vi "Main.vi"(8 "error in (no error)":T1) -> (0 "error out":T1)   [LabVIEW 2019, in "Log.lvlib"]
doc: "Logs commands and errors in\nlog file"
uses:
  Log.lvlib
  module data.ctl
  log module message.ctl
  <vilib>/Field R&D Services/Logger/Type Definitions/Severity.ctl
  681a73ac-a301-4c4f-9af0-9afa4de37740.vi
  Log GV.vi
  SubVIs/Shared/Comm GV.vi
  SubVIs/Shared/System GV.vi
  <vilib>/Field R&D Services/Logger/Support/Manager.vi
  <vilib>/Field R&D Services/Logger/Support/Control State.vi
  SubVIs/Shared/Shared.lvlib
  <vilib>/Field R&D Services/Logger/Field_RnD_Services_Logger_Toolkit.lvlib
panel:
  in  "stop wd":bool
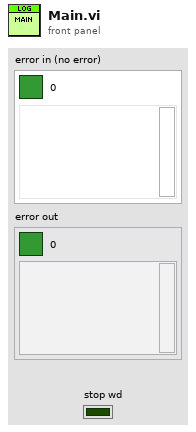
[diagram p1: front panel]
types:
  T1 = cluster{"Boolean Round":bool, "code":i32, "source":string}
  T2 = typedef "Log.lvlib/log module message.ctl" = cluster{"msg":string, "data":string}
  T3 = typedef "Log.lvlib/module data.ctl" = cluster{"dummy":dbl}
  T4 = typedef "Field_RnD_Services_Logger_Toolkit.lvlib/Severity.ctl" = enum16{"Benign", "Warning", "Recoverable", "Fatal"}
  T5 = typedef "CommandResponse communication.lvlib/Status + response + data cluster.ctl" = cluster{"message":string, "response":string, "data":variant}
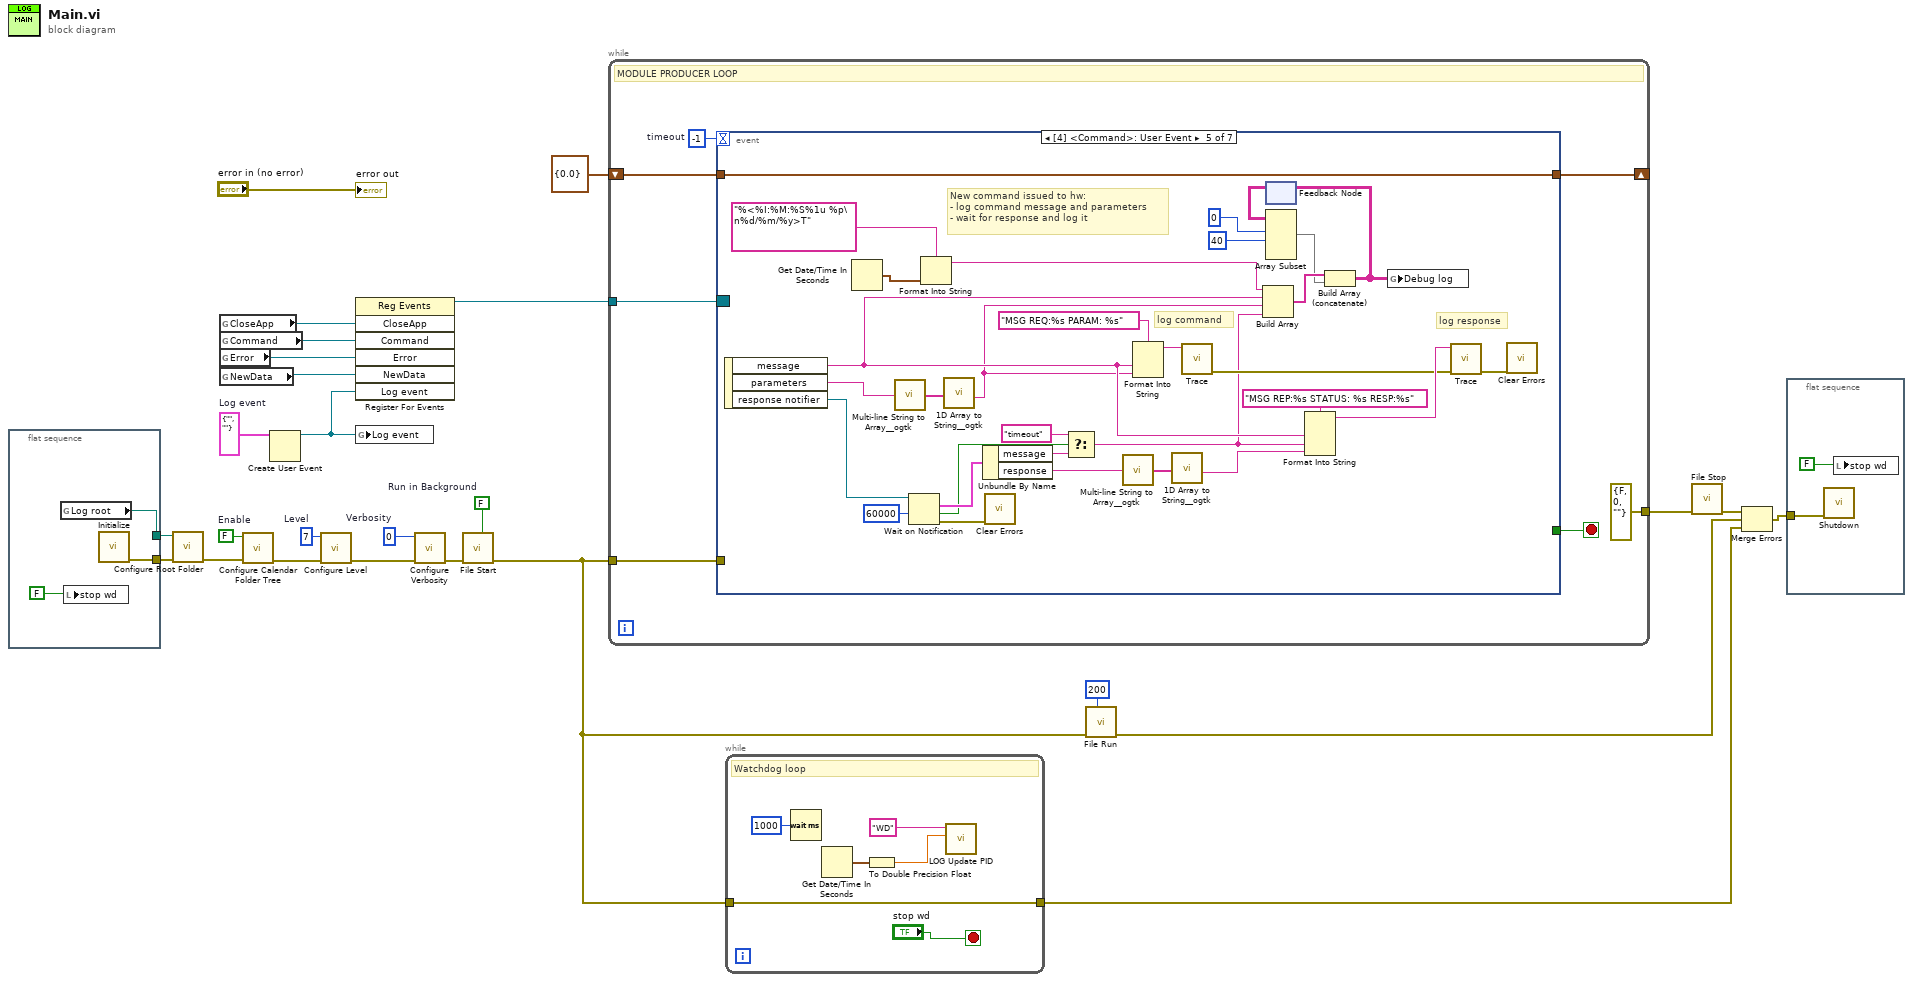
[diagram p0: block diagram]
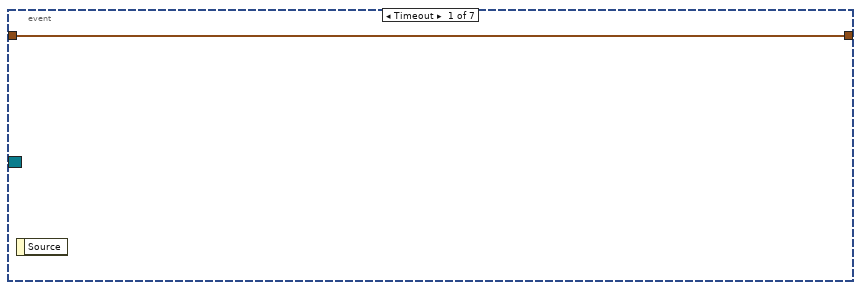
[diagram p2: hidden frame]
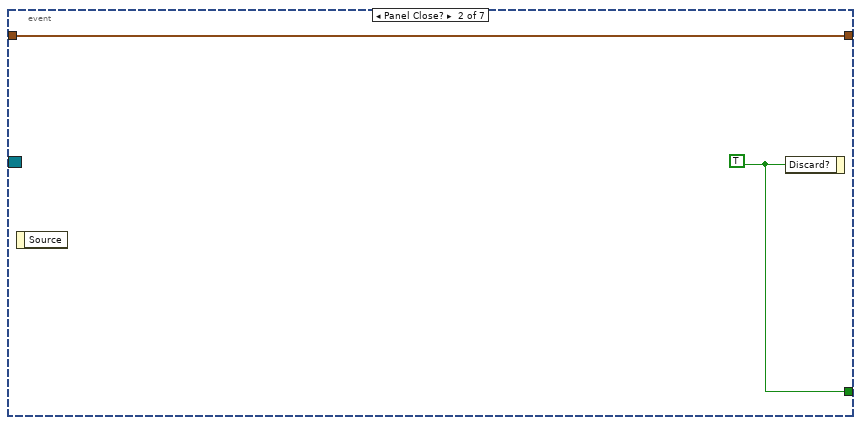
[diagram p3: hidden frame]
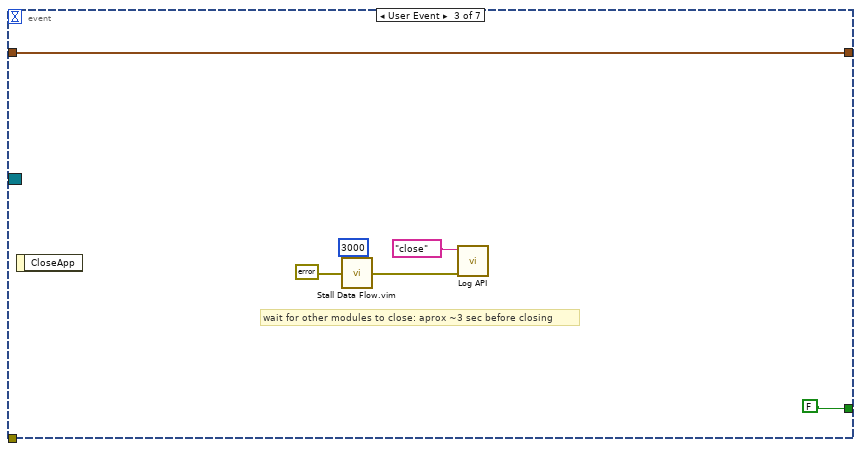
[diagram p4: hidden frame]
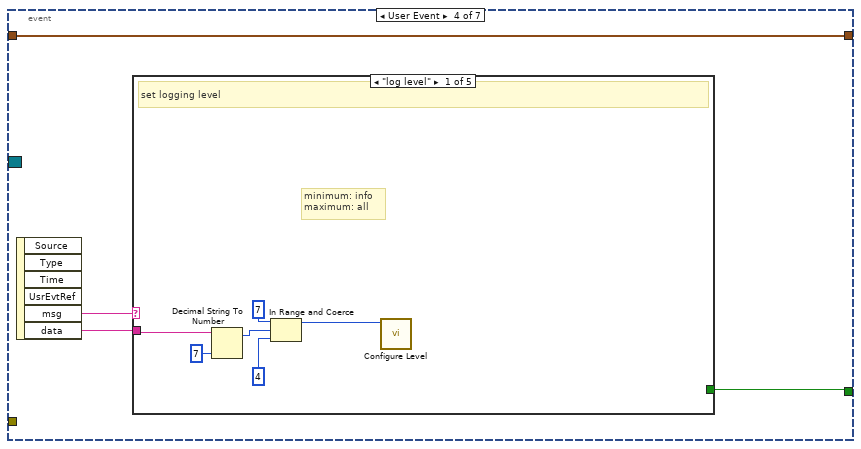
[diagram p5: hidden frame]
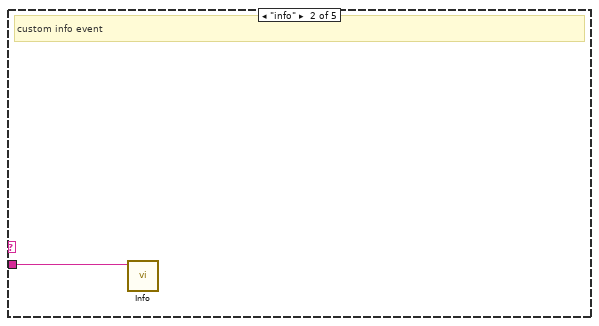
[diagram p6: hidden frame]
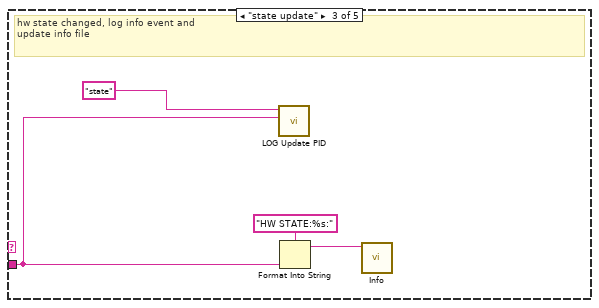
[diagram p7: hidden frame]
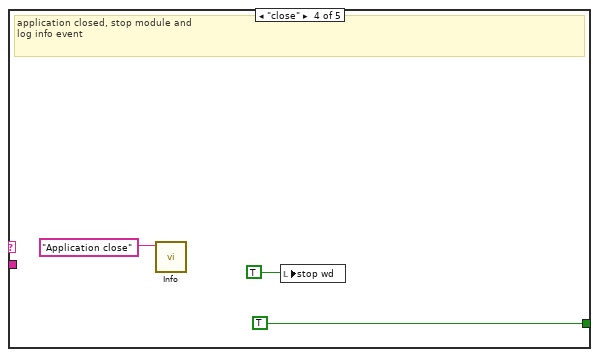
[diagram p8: hidden frame]
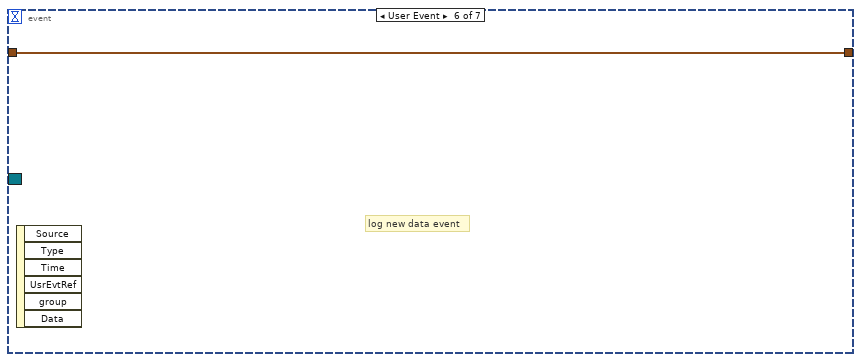
[diagram p10: hidden frame]
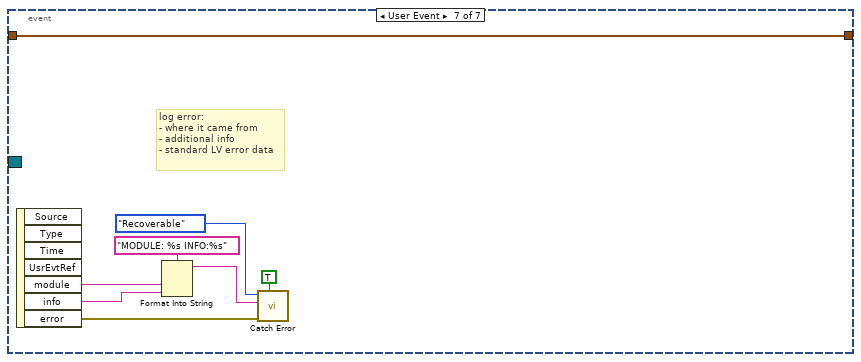
[diagram p11: hidden frame]
diagram:
  w5 = T2 {"msg"="", "data"=""}  # Log event
  w11 = u8 7  # Level
  w13 = FALSE  # Run in Background
  w17 = u8 0  # Verbosity
  w14 = FALSE  # Enable
  n1 = flat-sequence {
    tunnel: [w29] -> w20
    tunnel: [w28] -> w19
    frame #0 {
      n2 = global read "System GV.vi" "Log root"() -> (w28:path)
      n3 = local write "stop wd"(FALSE) -> ()
      n4 = call <vilib>:"Initialize.vi"() -> ("Error Out"=w29:errorcluster)  [unwired: 11 in]
    }
  }
  n5 = call <vilib>:"Configure Root Folder.vi"("Error In"=w20, "Root Folder"=w19) -> ("Error Out"=w12:errorcluster)  [unwired: 9 in]
  n6 = global read "Comm GV.vi" "CloseApp"() -> (w24:refnum<user-event>)
  n7 = global read "Comm GV.vi" "Command"() -> (w23:refnum<user-event>)
  n8 = global read "Comm GV.vi" "Error"() -> (w22:refnum<user-event>)
  n9 = global read "Comm GV.vi" "NewData"() -> (w21:refnum<user-event>)
  n10 = call <vilib>:"Configure Calendar Folder Tree.vi"("Error In"=w12, "Enable"=w14) -> ("Error Out"=w15:errorcluster)  [unwired: 9 in]
  n11 = Create User Event(user event datatype=w5) -> (user event=w4:refnum<user-event>)  [unwired: 1 in, 1 out]
  n12 = call <vilib>:"Configure Level.vi"("Error In"=w15, "Level"=w11) -> ("Error Out"=w18:errorcluster)  [unwired: 9 in]
  n13 = register-events(w24, w23, w22, w21, w4) -> (reference out=w26:refnum<event-registration>)  [unwired: 2 in, 1 out]
  n14 = global write "Log GV.vi" "Log event"(w4) -> ()
  n15 = call <vilib>:"Configure Verbosity.vi"("Error In"=w18, "Verbosity"=w17) -> ("Error Out"=w16:errorcluster)  [unwired: 9 in]
  n16 = call <vilib>:"File Start.vi"("Run in Background"=w13, "Error In"=w16) -> ("Error Out"=w2:errorcluster)  [unwired: 9 in]
  n17 = while {
    tunnel: w26 -> [w36]
    shift-right: [w33] -> _
    shift-left: T3 {"dummy"=0.0} ("module loopdata") -> [w34]
    tunnel: w2 -> [w31]
    tunnel: [errorcluster {"status"=FALSE, "code"=0, "source"=""} ("error constant")] -> w10
    stop <- w32 stop-if-true
    w35 = -1  # timeout
    # "MODULE PRODUCER LOOP"
    n18 = event shown="[4] <Command>: User Event" {
      selector: w36 -> [_ _ _ _ _ _ _]
      dyn-events: _ -> [_ _ _ _ _ _ _]
      timeout: w35 -> [_ _ _ _ _ _ _]
      tunnel: w34 -> [w37 w39 w45 w49 w94 w95 w103]
      tunnel: [w37 w39 w45 w49 w94 w95 w103] -> w33
      tunnel: [_ w38 FALSE w46 _ _ _] -> w32
      tunnel: w31 -> [_ _ _ _ _ _ _]
      event Timeout {
        n19 = event-data() -> ()  [unwired: 1 in, 1 out]
      }
      event Panel Close? {
        w38 = TRUE ("Discard?")
        n20 = event-data() -> ()  [unwired: 1 in, 1 out]
        n21 = event-data("Discard?"=w38) -> ()  [unwired: 1 in, 1 out]
      }
      event User Event {
        # "wait for other modules to close: aprox ~3 sec before closing"
        n22 = event-data() -> ()  [unwired: 1 in, 1 out]
        n23 = call "Stall Data Flow.vim"("value in"=errorcluster {"status"=FALSE, "code"=0, "source"=""} ("error constant"), "milliseconds to wait"=u32 3000) -> ("value out"=w42:errorcluster)  [unwired: 1 out]
        n24 = call "Log API.vi"("error in (no error)"=w42, "message"="close") -> ()  [unwired: 9 in, 1 out]
      }
      event User Event {
        n25 = event-data() -> ("msg"=w48:string, "data"=w47:string)  [unwired: 1 in, 4 out]
        n26 = case shown="\"log level\"" w48 {
          tunnel: w47 -> [w55 w56 w58 _ _]
          tunnel: [_ _ _ TRUE _] -> w46
          frame "log level" {
            # "minimum: info\nmaximum: all"
            # "set logging level"
            n27 = Decimal String To Number(string=w55, default (0L)=7 ("default (0 I32)")) -> (offset past number=w53:i32)  [unwired: 1 in, 1 out]
            n28 = In Range and Coerce(upper limit=7 ("default (0 I32)"), x=w53, lower limit=4 ("default (0 I32)")) -> (coerced(x)=w50:i32)  [unwired: 1 out]
            n29 = call <vilib>:"Configure Level.vi"("Level"=w50) -> ()  [unwired: 10 in, 1 out]
          }
          frame "info" {
            # "custom info event"
            n30 = call <vilib>:"Info.vi"("Message"=w56) -> ()  [unwired: 10 in, 1 out]
          }
          frame "state update" {
            # "hw state changed, log info event and\nupdate info file"
            n31 = call "LOG Update PID.vi"("data"=w58, "key"="state") -> ()  [unwired: 10 in]
            n32 = Format Into String(format string="HW STATE:%s:", w58) -> (resulting string=w60:string)  [unwired: 2 in, 1 out]
            n33 = call <vilib>:"Info.vi"("Message"=w60) -> ()  [unwired: 10 in, 1 out]
          }
          frame "close" {
            # "application closed, stop module and\nlog info event"
            n34 = call <vilib>:"Info.vi"("Message"="Application close") -> ()  [unwired: 10 in, 1 out]
            n35 = local write "stop wd"(TRUE) -> ()
          }
          frame Default {
          }
        }
      }
      event User Event {
        # "New command issued to hw:\n- log command message and parameters\n- wait for response and log it"
        # "log response"
        # "log command"
        n36 = event-data() -> ("message"=w75:string, "parameters"=w93:string, "response notifier"=w91:refnum<notifier>)  [unwired: 1 in]
        n37 = Get Date/Time In Seconds() -> (seconds since 1Jan1904=w66:timestamp)
        n38 = call <userlib>:"Multi-line String to Array__ogtk.vi"("string"=w93) -> ("lines"=w92:string[])
        n39 = Wait on Notification(notifier=w91, timeout in ms (-1)=60000) -> (notification=w88:T5, timed out?=w79:bool, error out=w89:errorcluster)  [unwired: 2 in, 1 out]
        n40 = Format Into String(format string="%<%I:%M:%S%1u %p\n%d/%m/%y>T", w66) -> (resulting string=w65:string)  [unwired: 2 in, 1 out]
        n41 = call <userlib>:"1D Array to String__ogtk.vi"("Array of Strings"=w92) -> ("delimited string"=w74:string)  [unwired: 10 in]
        n42 = Unbundle By Name(w88) -> ("message"=w78:string, "response"=w84:string)
        n43 = call <vilib>:"Clear Errors.vi"("error in (no error)"=w89) -> ()  [unwired: 5 in, 2 out]
        n44 = Select(t="timeout", s=w79, f=w78) -> (s? t:f=w73:string)
        n45 = call <userlib>:"Multi-line String to Array__ogtk.vi"("string"=w84) -> ("lines"=w85:string[])
        n46 = Format Into String(format string="MSG REQ:%s PARAM: %s", w75, w74) -> (resulting string=w86:string)  [unwired: 2 in, 1 out]
        n47 = call <userlib>:"1D Array to String__ogtk.vi"("Array of Strings"=w85) -> ("delimited string"=w82:string)  [unwired: 10 in]
        n48 = call <vilib>:"Trace.vi"("Message"=w86) -> ("Error Out"=w80:errorcluster)  [unwired: 10 in]
        n49 = Build Array(w65, w75, w74, w73) -> (w72:string[])
        n50 = feedback #1() -> (w71:string[][])  [unwired: 1 in]
        n51 = Array Subset(array=w71, index (row)=0 ("index"), length (row)=40 ("length")) -> (w68:string[][])  [unwired: 2 in]
        n52 = Format Into String(format string="MSG REP:%s STATUS: %s RESP:%s", w75, w73, w82) -> (resulting string=w81:string)  [unwired: 2 in, 1 out]
        n53 = Build Array (concatenate)(w72, w68) -> (w67:string[][])
        n54 = feedback-in #1(w67) -> ()
        n55 = global write "Log GV.vi" "Debug log"(w67) -> ()
        n56 = call <vilib>:"Trace.vi"("Error In"=w80, "Message"=w81) -> ("Error Out"=w76:errorcluster)  [unwired: 9 in]
        n57 = call <vilib>:"Clear Errors.vi"("error in (no error)"=w76) -> ()  [unwired: 5 in, 2 out]
      }
      event User Event {
        # "log new data event"
        n58 = event-data() -> ()  [unwired: 1 in, 6 out]
      }
      event User Event {
        # "log error:\n- where it came from\n- additional info\n- standard LV error data"
        n59 = event-data() -> ("module"=w98:string, "info"=w97:string, "error"=w101:T1)  [unwired: 1 in, 4 out]
        n60 = Format Into String(format string="MODULE: %s INFO:%s", w98, w97) -> (resulting string=w100:string)  [unwired: 2 in, 1 out]
        n61 = call <vilib>:"Catch Error.vi"("Clear"=TRUE, "Error In"=w101, "Source"=w100, "Severity"=Severity."Recoverable") -> ()  [unwired: 7 in, 1 out]
      }
    }
  }
  n62 = while {
    tunnel: w2 -> [w104]
    tunnel: [w104] -> w1
    stop <- "stop wd" stop-if-true
    # "Watchdog loop"
    n63 = Wait (ms)(milliseconds to wait=u32 1000) -> ()  [unwired: 1 out]
    n64 = Get Date/Time In Seconds() -> (seconds since 1Jan1904=w106:timestamp)
    n65 = To Double Precision Float(number=w106) -> (double precision float=w105:dbl)
    n66 = call "LOG Update PID.vi"("data"=w105, "key"="WD") -> ()  [unwired: 10 in]
  }
  n67 = call <vilib>:"File Run.vi"("Write Period"=u32 200, "Error In"=w2) -> ("Error Out"=w7:errorcluster)  [unwired: 9 in]
  n68 = call <vilib>:"File Stop.vi"("Error In"=w10) -> ("Error Out"=w9:errorcluster)  [unwired: 10 in]
  n69 = Merge Errors(w9, w7, w1) -> (w8:errorcluster)
  n70 = flat-sequence {
    tunnel: w8 -> [w111]
    frame #0 {
      n71 = call <vilib>:"Shutdown.vi"("Error In"=w111) -> ()  [unwired: 10 in, 1 out]
      n72 = local write "stop wd"(FALSE) -> ()
    }
  }
  "error out" <- "error in (no error)"
